vi "Get or Init Class.vi"(7 "target PDE":refnum<class "NI_PDE.lvclass">, 8 "error in (no error)":errorcluster, 11 "PDE in":refnum<class "NI_PDE.lvclass">) -> (0 "error out":errorcluster, 3 "PDE out":refnum<class "NI_PDE.lvclass">)   [LabVIEW 2017, in "NI_PDE.lvlib" / "NI_PDE.lvclass"]
uses:
  <vilib>/gmath/pde.llb/PDEClass/NI_PDE.lvclass
  <vilib>/gmath/pde.llb/PDEClass/Class Type.ctl
  <vilib>/gmath/pde.llb/Common/PDE_Error.ctl
  <vilib>/gmath/NI_PDE.lvlib
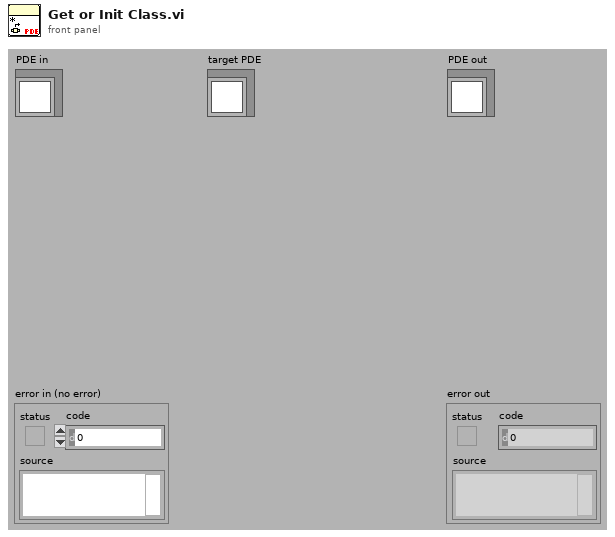
[diagram p1: front panel]
types:
  T1 = typedef "NI_PDE.lvlib/PDE_Error.ctl" = enum16{"No Error", "k is zero", "End point <= start point", "# of time steps < 2", "# of spatial points < 3", "# of grid < 1 for FEM", "# of boundary < 3 for FEM", "Incompatible RHS size", "Incompatible BC size", "Incompatible IC size", "PDE class conflict", "RHS class conflict", "Domain class conflict", "BC class conflict", "IC class conflict"}
  T2 = typedef "NI_PDE.lvlib/NI_PDE.lvclass/Class Type.ctl" = i32
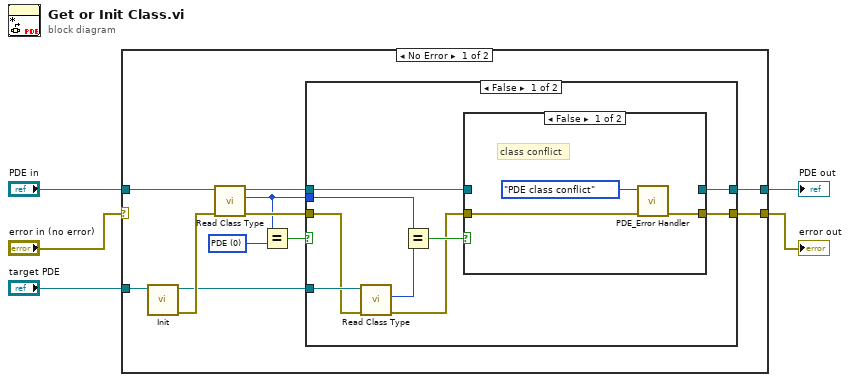
[diagram p0: block diagram]
diagram:
  n1 = case shown="No Error" "error in (no error)" {
    selector: "error in (no error)" -> [_ w34]
    tunnel: "PDE in" -> [w16 w33]
    tunnel: [w10 w33] -> w4
    tunnel: [w9 w34] -> w3
    tunnel: "target PDE" -> [w8 _]
    frame No Error {
      w15 = T2 0 items=["PDE"=0, "PDE_2ndOrder_ConstPara"=100, "PDE_Helmholtz_2D"=112, "PDE_Heat_1D"=121, "PDE_Heat_2D"=122, "PDE_Wave_1D"=131, "PDE_Wave_2D"=132] ("y")
      n2 = call-dynamic "Init.vi"("PDE"=w8) -> ("error out"=w7:errorcluster, "initialized PDE"=w6:refnum<class "NI_PDE.lvclass">)  [unwired: 1 in, 8 out]
      n3 = call-dynamic "Read Class Type.vi"("error in (no error)"=w7, "PDE.lvclass in"=w16) -> ("error out"=w12:errorcluster, "PDE class type"=w11:T2, "PDE.lvclass out"=w13:refnum<class "NI_PDE.lvclass">)  [unwired: 7 out]
      n4 = Equal?(x=w11, y=w15) -> (x = y?=w14:bool)
      n5 = case shown="False" w14 {
        tunnel: w13 -> [w24 _]
        tunnel: w12 -> [w18 w31]
        tunnel: [w23 w32] -> w10
        tunnel: [w22 w31] -> w9
        tunnel: w11 -> [w25 _]
        tunnel: w6 -> [w20 w32]
        frame False {
          n6 = call-dynamic "Read Class Type.vi"("error in (no error)"=w18, "PDE.lvclass in"=w20) -> ("error out"=w17:errorcluster, "PDE class type"=w19:T2)  [unwired: 8 out]
          n7 = Equal?(x=w25, y=w19) -> (x = y?=w21:bool)
          n8 = case shown="False" w21 {
            tunnel: w24 -> [_ w29]
            tunnel: [_ w29] -> w23
            tunnel: [w28 w30] -> w22
            tunnel: w17 -> [w27 w30]
            frame False {
              # "class conflict"
              n9 = call <vilib>:"PDE_Error Handler.vi"("error in (no error)"=w27, "PDE error"=PDE_Error."PDE class conflict") -> ("error out"=w28:errorcluster)  [unwired: 9 out]
            }
            frame True {
            }
          }
        }
        frame True {
        }
      }
    }
    frame Error {
    }
  }
  "PDE out" <- w4
  "error out" <- w3
